vi "map_controller.vi"(0 "eps":dbl, 2 "redy":dbl[](array[numeric]), 3 "redx":dbl[](array[numeric]), 4 "bluex":dbl[](array[numeric]), 5 "yellowx":dbl[](array[numeric]), 6 "bluey":dbl[](array[numeric]), 7 "yellowy":dbl[](array[numeric]), 8 "pos":dbl[](array[numeric]), 9 "vec":dbl[](array[numeric]), 10 "orangey":dbl[](array[numeric]), 11 "orangex":dbl[](array[numeric])) -> (1 "Map object out":cluster{"orangex":dbl[], "orangey":dbl[]}[](array[cluster]))   [LabVIEW 2017]
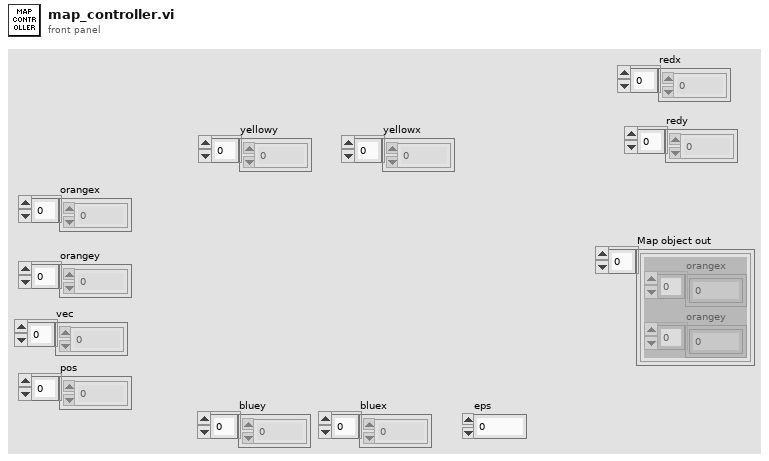
[diagram p1: front panel]
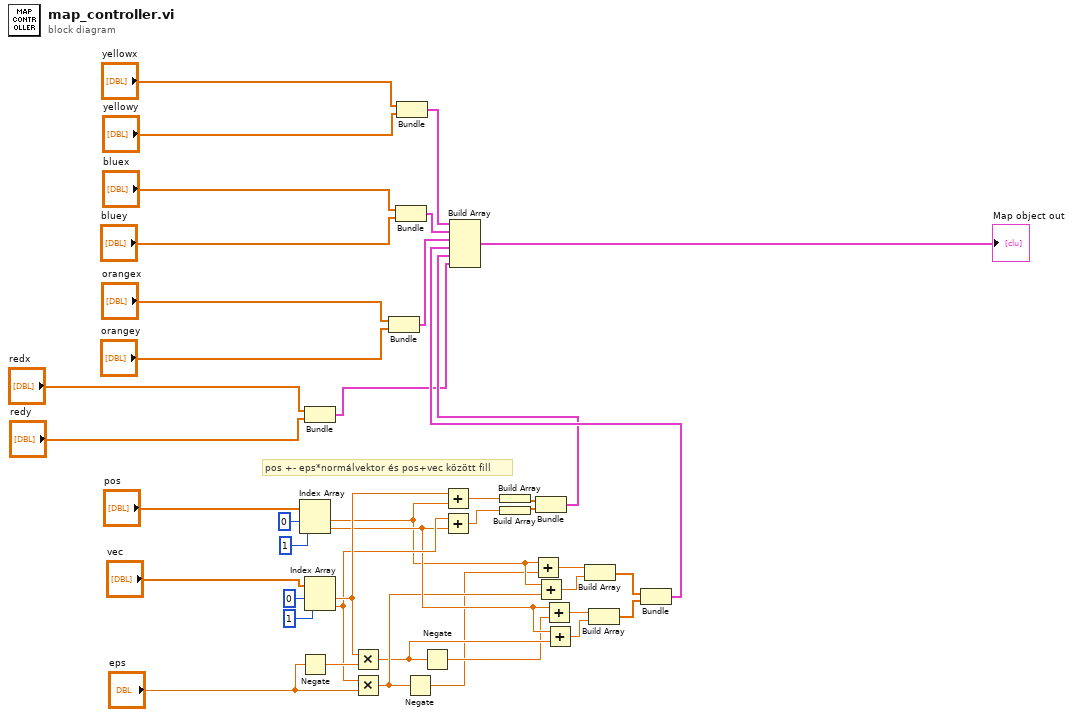
[diagram p0: block diagram]
diagram:
  # "pos +- eps*normálvektor és pos+vec között fill"
  n1 = Index Array(array="pos", index #1=0 ("index"), index #2=1 ("index")) -> (element #1=w13:dbl, element #2=w15:dbl)
  n2 = Negate(x="eps") -> (-x=w39:dbl)
  n3 = Bundle("redx"="redx", "redy"="redy") -> (w1:cluster{"redx":dbl[], "redy":dbl[]})  [unwired: 1 in]
  n4 = Index Array(array="vec", index #1=0 ("index"), index #2=1 ("index")) -> (element #1=w18:dbl, element #2=w17:dbl)
  n5 = Multiply(x=w18, y=w39) -> (x*y=w11:dbl)
  n6 = Multiply(x=w17, y="eps") -> (x*y=w12:dbl)
  n7 = Bundle("orangex"="orangex", "orangey"="orangey") -> (w4:cluster{"orangex":dbl[], "orangey":dbl[]})  [unwired: 1 in]
  n8 = Bundle("bluex"="bluex", "bluey"="bluey") -> (w5:cluster{"bluex":dbl[], "bluey":dbl[]})  [unwired: 1 in]
  n9 = Bundle("yellowx"="yellowx", "yellowy"="yellowy") -> (w6:cluster{"yellowx":dbl[], "yellowy":dbl[]})  [unwired: 1 in]
  n10 = Negate(x=w12) -> (-x=w9:dbl)
  n11 = Negate(x=w11) -> (-x=w10:dbl)
  n12 = Add(x=w18, y=w13) -> (x+y=w22:dbl)
  n13 = Add(x=w17, y=w15) -> (x+y=w21:dbl)
  n14 = Build Array(w22) -> (w24:dbl[])
  n15 = Build Array(w21) -> (w23:dbl[])
  n16 = Add(x=w13, y=w9) -> (x+y=w14:dbl)
  n17 = Bundle(w24, w23) -> (w2:cluster{dbl[], dbl[]})  [unwired: 1 in]
  n18 = Add(x=w13, y=w12) -> (x+y=w20:dbl)
  n19 = Add(x=w15, y=w10) -> (x+y=w16:dbl)
  n20 = Add(x=w15, y=w11) -> (x+y=w19:dbl)
  n21 = Build Array(w14, w20) -> (w41:dbl[])
  n22 = Build Array(w16, w19) -> (w26:dbl[])
  n23 = Bundle(w41, w26) -> (w3:cluster{dbl[], dbl[]})  [unwired: 1 in]
  n24 = Build Array(w6, w5, w4, w3, w2, w1) -> (→"Map object out":cluster{"redx":dbl[], "redy":dbl[]}[])
